vi "3_1_Face_Detection_Inference(CPU,GPU,RT)(Cam).vi"() -> ()   [LabVIEW 2020]
doc: "This example demonstrates the usage of the \"DeepLTK FPGA Addon\" for deploying a Face Detection model on a PXI-FPGA board, utilizing an input image sourced from a camera. \n\nMore Examples: https://github.com/ngenehub/deepltk_fpga_examples"
uses:
  <vilib>/Ngene/Deep Learning Toolkit/Toolkit/NN_Network/Controls/NN_Device.ctl
  <vilib>/vision/driver/IMAQdx.llb/IMAQdx Camera Control Mode.ctl
  <vilib>/Ngene/Deep Learning Toolkit/Toolkit/NN_Network/Controls/NN_Save_Before_Destroy_Options.ctl
  <vilib>/vision/driver/IMAQdx.llb/IMAQdx Buffer Number Mode.ctl
  94985df4-208a-4d6b-b1ec-530e3fcff878.vi
  <vilib>/Ngene/Deep Learning Toolkit/Toolkit/NN_Network/API/NN_Set_Input/3D/NN_Set_Input(3D_SGL_idx).vi
  <vilib>/Ngene/Deep Learning Toolkit/Toolkit/Deep_Learning_Toolkit_by_Ngene.lvlib
  <vilib>/vision/NI_Vision_Development_Module.lvlib
  <vilib>/vision/driver/NI_Vision_Acquisition_Software.lvlib
  <resource>/objmgr/imaqdx.rc
  <vilib>/ptbypt/NI_PtbyPt.lvlib
panel:
  in  "NN_Device":T1
  out "Inference time":dbl=0.10057269999997516 format="%#_4p"
  out "Loop time":dbl=0.10057269999997516 format="%#_4p"
  in  "Camera Resolution":i32(listbox)
  out "Display":T2(plugin-control)
  in  "Confidence_Thresh":sgl=0.19999999
  in  "IOU_Thresh":sgl=0.3
  in  "Camera":refnum<k21>="cam0" caption="IMAQdx Session"
  in  "Weight File Path":path=path "D:/Ngene/GitHub/deepltk_fpga_examples/2_Face_Detection(PXI,sbRIO)/Models/Face_Detection_Original/Face_Detection.bin"
  in  "Configuration File Path":path=path "D:/Ngene/GitHub/deepltk_fpga_examples/2_Face_Detection(PXI,sbRIO)/Models/Face_Detection_Original/Face_Detection.cfg"
  in  "Stop":bool
  # "Overview:  This example demonstrates usage of Deep Learning Toolkit for deploying a Face Detection model, utilizing an input image sourced from a camera.\nThis VI can also be executed on RT targets.\nRequirements: \n•DeepLTK - Deep Learning Toolkit for LabVIEW (https://www.ngene.co/deep-learning-toolkit-for-labview)\n• NI Vision Development Module\n• Web Camera"
  # "Instructions:\nNote: To run the example on an RT target, copy the pretrained model to the RT target.\n1. Provide the \"Network Configuration File Path\" and \"Weight File Path\" locted in \"Models\\Face_Detection_Original\" folder in the project.\n2.\tSelect the camera from \"Camera\" control.\n3.\tUse NN_Device to specify the device (CPU or GPU) for execution. GPU is applicable only for 64-bit LabVIEW.\n4.\tRun the VI. \n5.\t Observe the detections drawn on the \"Display\". The info on the top left of each bounding box represents detected object class and the confidence level.  \n \nMore Examples: https://github.com/ngenehub/deepltk_fpga_examples"
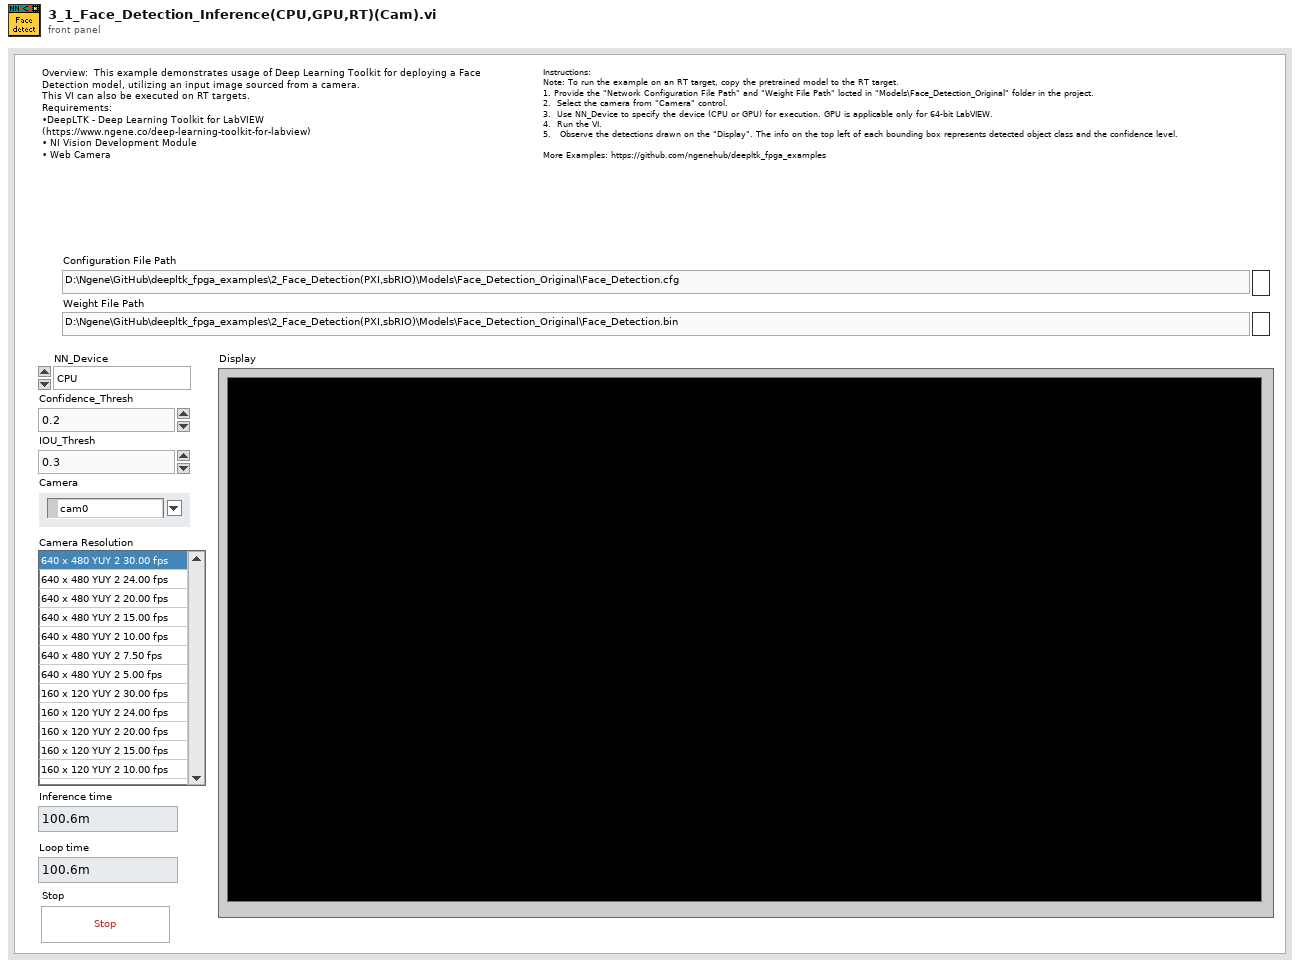
[diagram p1: front panel]
types:
  T1 = typedef "Deep_Learning_Toolkit_by_Ngene.lvlib/NN_Device.ctl" = enum16{"CPU", "GPU"}
  T2 = typedef "IMAQ Image.ctl" = refnum<image>
  T3 = typedef "Deep_Learning_Toolkit_by_Ngene.lvlib/NN_Save_Before_Destroy_Options.ctl" = cluster{"CFG?":bool, "Weights?":bool, "Render?":bool}
  T4 = typedef "NI_Vision_Acquisition_Software.lvlib/IMAQdx Camera Control Mode.ctl" = enum32{"Controller", "Listener"}
  T5 = typedef "Image Type" = u32
  T6 = typedef "IMAQdx.ctl" = refnum<k21>
  T7 = typedef "Deep_Learning_Toolkit_by_Ngene.lvlib/NN_Config_Params.ctl" = cluster{"Name":string, "mBatch":i32, "NN_Train_Params":T8, "LR_Decay_Policy":T11, "Labels":string[], "Loss":T13}
  T8 = typedef "Deep_Learning_Toolkit_by_Ngene.lvlib/NN_Train_Params.ctl" = cluster{"Optimizer":T9, "Beta_1":sgl, "Beta_2":sgl, "Weight Decay(L1)":sgl, "Weight Decay(L2)":sgl, "Data_Sampling":T10}
  T9 = typedef "Deep_Learning_Toolkit_by_Ngene.lvlib/NN_Train_Optimizer.ctl" = enum16{"SGD", "Adam", "Adagrad", "Adadelta", "RMSProp", "Nesterov"}
  T10 = typedef "Deep_Learning_Toolkit_by_Ngene.lvlib/NN_Train_Data_Sampling.ctl" = enum16{"Random", "Sequential"}
  T11 = typedef "Deep_Learning_Toolkit_by_Ngene.lvlib/NN_LR_Policy_Cfg.ctl" = cluster{"Policy_Type":T12, "LR0":dbl, "k":sgl, "WarmUp_Policy":enum16{"Step", "Ramp"}, "WarmUp_Iter":i32, "WarmUp_Ratio":sgl}
  T12 = typedef "Deep_Learning_Toolkit_by_Ngene.lvlib/NN_LR_Policy_Type.ctl" = enum16{"Manual", "Step", "Exp", "1/t"}
  T13 = typedef "Deep_Learning_Toolkit_by_Ngene.lvlib/NN_Loss_Config_Params.ctl" = cluster{"Loss_Type":T14, "Loss_Conf_Params":variant}
  T14 = typedef "Deep_Learning_Toolkit_by_Ngene.lvlib/NN_Loss_Type.ctl" = enum16{"None", "MSE", "CrossEntropy", "YOLO_v2", "YOLO_v4"}
  T15 = typedef "Deep_Learning_Toolkit_by_Ngene.lvlib/NN_Layer_Config_Params.ctl" = cluster{"Layer_Type":T16, "Layer_Conf_Params":variant, "Input Layers":string[]}
  T16 = typedef "Deep_Learning_Toolkit_by_Ngene.lvlib/NN_Layer_Type.ctl" = enum16{"Input1D", "Input3D", "Conv1D", "Conv2D", "Conv2D_Adv", "MaxPool", "AvgPool", "UpSample", "DropOut3D", "ShortCut", "Concat", "SoftMax3D", "FC", "DropOut", "Softmax", "Flatten", "YOLO_v2", "YOLO_v4", "Activation", "BatchNormalization", "Unsupported"}
  T17 = typedef "Deep_Learning_Toolkit_by_Ngene.lvlib/NN.ctl" = cluster{"Name":string, "No of Layers":i32, "mBatch":i32, "Layers":T18[], "Dimty":T19, "Dims_In":T20, "Dims_Out":T20, "Working_Dir":path, "Train?":bool, "Train_Params":T8, "LR_Update_Policy":T11, "Session Data":T21, "Ground_truth":T22, "NNg_hdls":T23, "NN_Device":T1, "GPU Id":i32, "Labels":string[], "Receptive Field":T24[], "Loss_Type":T14, "Loss_Cfg_Prms":variant, "NNG_WS":T25}
  T18 = typedef "Deep_Learning_Toolkit_by_Ngene.lvlib/NN_Layer_ref.ctl" = refnum<data-value>
  T19 = typedef "Deep_Learning_Toolkit_by_Ngene.lvlib/NN_In_Out_Dim-ty.ctl" = enum8{"In1D_Out1D", "In3D_Out1D", "In3D_Out3D", "In3D_OutBBox"}
  T20 = typedef "Deep_Learning_Toolkit_by_Ngene.lvlib/NN_Dims(C,H,W).ctl" = cluster{"C":i32, "H":i32, "W":i32}
  T21 = typedef "Deep_Learning_Toolkit_by_Ngene.lvlib/NN_Train_Session_Data.ctl" = cluster{"Epochs":sgl, "Tot_Iter":i32, "LR":sgl, "LR_iter":i32}
  T22 = typedef "Deep_Learning_Toolkit_by_Ngene.lvlib/NN_Ground_truth.ctl" = cluster{"Y":variant}
  T23 = typedef "Deep_Learning_Toolkit_by_Ngene.lvlib/nng_cuda_handles.ctl" = cluster{"cudnn":u64, "cublas":u64, "stream":u64, "curand":u64}
  T24 = typedef "Deep_Learning_Toolkit_by_Ngene.lvlib/NN_Dims(V,H).ctl" = cluster{"V":i32, "H":i32}
  T25 = typedef "Deep_Learning_Toolkit_by_Ngene.lvlib/NNG_WS.ctl" = cluster{"NNG_WS_Mem":T26, "Max_WS_Size":i64}
  T26 = typedef "Deep_Learning_Toolkit_by_Ngene.lvlib/NNg_WS_Mem_DVR.ctl" = refnum<data-value>
  T27 = typedef "NI_Vision_Acquisition_Software.lvlib/IMAQdx Buffer Number Mode.ctl" = enum32{"Next", "Last", "Buffer Number", "Every", "Last New"}
  T28 = typedef "Deep_Learning_Toolkit_by_Ngene.lvlib/NN_Layer.ctl" = cluster{"Name":string, "Layer_Data":variant, "Layer_Type":T16, "Dims_In":T20, "Layers_In":variant, "Dims_Out":T20, "Layers_Out":variant, "Metrics":T29, "GPU_Data":variant, "mBatch":i32, "NN_Device":T1, "NNg_hdls":T23, "Train?":bool, "Dimty":T30, "RecptField":T31}
  T29 = typedef "Deep_Learning_Toolkit_by_Ngene.lvlib/NN_Layer_Metrics.ctl" = cluster{"Data":dbl, "Params":dbl, "Ops":dbl}
  T30 = typedef "Deep_Learning_Toolkit_by_Ngene.lvlib/NN_Layer_Dimty.ctl" = enum16{"1D", "3D"}
  T31 = typedef "Deep_Learning_Toolkit_by_Ngene.lvlib/NN_Layer_RF_State.ctl" = cluster{"Dims":T24, "J":T24}
  T32 = typedef "Deep_Learning_Toolkit_by_Ngene.lvlib/NN_BBox_Detection.ctl" = cluster{"Class":i32, "Conf Level":sgl, "BBox":T33}
  T33 = typedef "Deep_Learning_Toolkit_by_Ngene.lvlib/NN_BBox.ctl" = cluster{"x":sgl, "y":sgl, "w":sgl, "h":sgl}
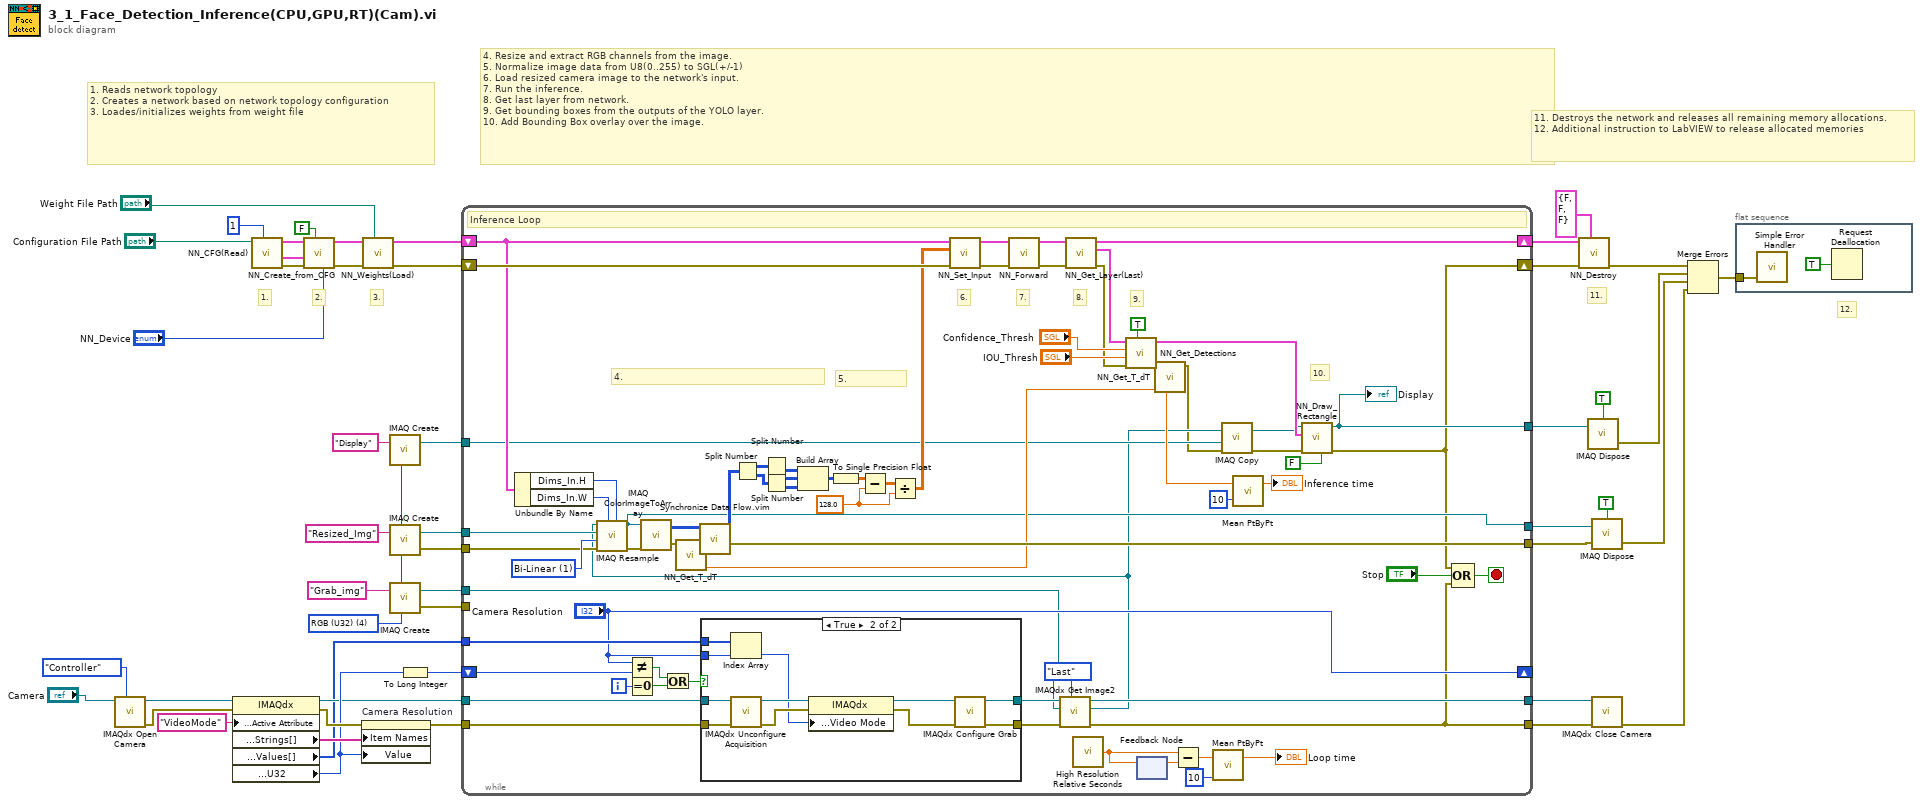
[diagram p0: block diagram]
diagram:
  w2 = T5 4 items=["Grayscale (U8)", "Grayscale (I16)", "Grayscale (SGL)", "Complex (CSG)", "RGB (U32)", "HSL (U32)", "RGB (U64)", "Grayscale (U16)"] ("Image Type")
  # "12."
  # "11.\tDestroys the network and releases all remaining memory allocations.\n12.\tAdditional instruction to LabVIEW to release allocated memories"
  # "11."
  # "4.\tResize and extract RGB channels from the image.\n5.\tNormalize image data from U8(0..255) to SGL(+/-1)\n6.\tLoad resized camera image to the network's input.\n7.\tRun the inference.\n8.\tGet last layer from network.\n9.\tGet bounding boxes from the outputs of the YOLO layer. \n10.\tAdd Bounding Box overlay over the image."
  # "1.\tReads network topology\n2.\tCreates a network based on network topology configuration\n3.\tLoades/initializes weights from weight file"
  # "3."
  # "2."
  # "1."
  n1 = call <vilib>:"IMAQdx Open Camera.vi"("Camera Control Mode"=IMAQdx_Camera_Control_Mode."Controller", "Session In"="Camera") -> ("error out"=w26:errorcluster, "Session Out"=w28:T6)  [unwired: 1 in, 7 out]
  n2 = property class="IMAQdx"(reference=w28, error in=w26, "Camera Attributes:Active Attribute"="VideoMode" ("ActiveAttribute")) -> (reference out=w22:T6, error out=w25:errorcluster, "Camera Attributes:Enum:Strings[]"=w24:string[], "Camera Attributes:Enum:Values[]"=w20:u32[], "Camera Attributes:Value:U32"=w23:u32)
  n3 = call <vilib>:"NN_CFG(Read).vi"("mBatch"=1, "CFG file path"="Configuration File Path") -> ("error out"=w46:errorcluster, "Net_Cfg"=w13:T7, "Layer_Cfg"=w47:T15[])  [unwired: 7 in]
  n4 = call <vilib>:"NN_Create_from_CFG.vi"("NN_Device"="NN_Device", "Train? (false)"=FALSE ("Train?"), "error in (no error)"=w46, "Net_Cfg"=w13, "Layer_Cfg"=w47) -> ("error out"=w45:errorcluster, "NN out"=w44:T17)  [unwired: 5 in]
  n5 = property on="Camera Resolution" class="LstBox (strict)"(error in=w25, "Item Names"=w24, "Value"=w23) -> (error out=w19:errorcluster)  [unwired: 1 in, 1 out]
  n6 = call <vilib>:"NN_Weights(Load).vi"("Weight File Path"="Weight File Path", "error in (no error)"=w45, "NN in"=w44) -> ("error out"=w8:errorcluster, "NN out"=w9:T17)  [unwired: 7 in]
  n7 = call "IMAQ Create"("Image Name"="Display", "Image Type"=w2) -> ("New Image"=w1:T2)  [unwired: 3 in, 1 out]
  n8 = call "IMAQ Create"("Image Name"="Resized_Img", "Image Type"=w2) -> ("New Image"=w34:T2, "error out"=w33:errorcluster)  [unwired: 3 in]
  n9 = call "IMAQ Create"("Image Name"="Grab_img", "Image Type"=w2) -> ("New Image"=w38:T2, "error out"=w41:errorcluster)  [unwired: 3 in]
  n10 = To Long Integer(number=w23) -> (32bit integer=w17:i32)
  n11 = while {
    shift-right: [w87] -> w39
    shift-left: w9 -> [w109]
    shift-right: [w49] -> w40
    shift-left: w8 -> [w114]
    tunnel: [w58] -> w42
    tunnel: w41 -> [_]
    tunnel: w38 -> [w54]
    tunnel: w34 -> [w110]
    tunnel: w33 -> [w100]
    tunnel: [w71] -> w32
    tunnel: [w60] -> w31
    tunnel: w22 -> [w98]
    tunnel: [w97] -> w21
    tunnel: w20 -> [w92]
    tunnel: w19 -> [w91]
    shift-right: ["Camera Resolution"] -> _
    shift-left: w17 -> [w90]
    tunnel: [w82] -> w11
    tunnel: w1 -> [w56]
    i -> [w88]
    stop <- w116 stop-if-true
    w74 = sgl 128.0
    w111 = u32 1 items=["Zero Order", "Bi-Linear", "Quadratic", "Cubic Spline"] ("Interpolation Type")
    # "10."
    # "9."
    # "8."
    # "7."
    # "6."
    # "4."
    # "5."
    # "Inference Loop"
    n12 = Unbundle By Name(w109) -> ("Dims_In.H"=w108:i32, "Dims_In.W"=w107:i32)
    n13 = Not Equal?(x="Camera Resolution", y=w90) -> (x != y?=w95:bool)
    n14 = Equal To 0?(x=w88) -> (x = 0?=w94:bool)
    n15 = Or(x=w95, y=w94) -> (x .or. y?=w96:bool)
    n16 = case shown="True" w96 {
      tunnel: w98 -> [w120 w129]
      tunnel: w91 -> [w119 w128]
      tunnel: [w120 w125] -> w93
      tunnel: [w119 w126] -> w53
      tunnel: w92 -> [_ w131]
      tunnel: "Camera Resolution" -> [_ w130]
      frame False {
      }
      frame True {
        n17 = Index Array(array=w131, index=w130) -> (element=w121:u32)
        n18 = call <vilib>:"IMAQdx Unconfigure Acquisition.vi"("error in"=w128, "Session In"=w129) -> ("error out"=w122:errorcluster, "Session Out"=w127:T6)  [unwired: 8 out]
        n19 = property class="IMAQdx"(reference=w127, error in=w122, "Acquisition Attributes:Video Mode"=w121) -> (reference out=w124:T6, error out=w123:errorcluster)
        n20 = call <vilib>:"IMAQdx Configure Grab.vi"("error in"=w123, "Session In"=w124) -> ("error out"=w126:errorcluster, "Session Out"=w125:T6)  [unwired: 2 in, 6 out]
      }
    }
    n21 = call <vilib>:"IMAQdx Get Image2.vi"("Buffer Number Mode (Next)"=IMAQdx_Buffer_Number_Mode."Last", "error in"=w53, "Image In"=w54, "Session In"=w93) -> ("error out"=w82:errorcluster, "Image Out"=w52:T2, "Session Out"=w97:T6)  [unwired: 4 in, 1 out]
    n22 = call "IMAQ Resample"("X Resolution"=w108, "Y Resolution"=w107, "error in (no error)"=w100, "Interpolation Type"=w111, "Image Dst"=w110, "Image Src"=w52) -> ("error out"=w99:errorcluster, "Image Dst Out"=w60:T2)  [unwired: 4 in]
    n23 = call "IMAQ ColorImageToArray"("Image"=w60, "error in (no error)"=w99) -> ("Image Pixels (U32)"=w73:u32[][], "error out"=w72:errorcluster)  [unwired: 2 in, 1 out]
    n24 = call <vilib>:"NN_Get_T_dT.vi"("error in (no error)"=w72) -> ("T_out"=w66:dbl, "error out"=w70:errorcluster)  [unwired: 6 in, 1 out]
    n25 = call "Synchronize Data Flow.vim"("input 3"=w70, "input 1"=w73) -> ("output 3"=w71:errorcluster, "output 1"=w69:u32[][])  [unwired: 2 in, 2 out]
    n26 = Split Number(x=w69) -> (hi(x)=w102:u16[][], lo(x)=w101:u16[][])
    n27 = Split Number(x=w102) -> (lo(x)=w103:u8[][])  [unwired: 1 out]
    n28 = Split Number(x=w101) -> (hi(x)=w104:u8[][], lo(x)=w105:u8[][])
    n29 = Build Array(w103, w104, w105) -> (w106:u8[][][])
    n30 = To Single Precision Float(number=w106) -> (single precision float=w79:sgl[][][])
    n31 = Subtract(x=w79, y=w74) -> (x-y=w84:sgl[][][])
    n32 = Divide(x=w84, y=w74) -> (x/y=w75:sgl[][][])
    n33 = call-poly <vilib>:"NN_Set_Input.vi"("error in (no error)"=w114, "Data_In(3D_SGL)"=w75, "NN in"=w109) -> ("error out"=w112:errorcluster, "NN out"=w113:T17)  [unwired: 7 in]
    n34 = call <vilib>:"NN_Forward.vi"("error in (no error)"=w112, "NN in"=w113) -> ("error out"=w85:errorcluster, "NN out"=w86:T17)  [unwired: 6 in, 2 out]
    n35 = call <vilib>:"NN_Get_Layer(Last).vi"("error in (no error)"=w85, "NN in"=w86) -> ("error out"=w68:errorcluster, "Last_Layer"=w83:T28, "NN out"=w87:T17)  [unwired: 6 in, 1 out]
    n36 = call <vilib>:"High Resolution Relative Seconds.vi"() -> ("relative seconds"=w117:dbl)
    n37 = call <vilib>:"NN_Get_Detections.vi"("Temporal Averaging (F)"=TRUE ("Enable Averaging"), "error in"=w68, "IOU_Thrsh"="IOU_Thresh", "Confidence_Thrsh"="Confidence_Thresh", "YOLO_Layer"=w83) -> ("error out"=w67:errorcluster, "Detections"=w80:T32[])  [unwired: 5 in]
    n38 = feedback #1() -> (w118:dbl)  [unwired: 1 in]
    n39 = feedback-in #1(w117) -> ()
    n40 = call <vilib>:"NN_Get_T_dT.vi"("T_in"=w66, "error in (no error)"=w67) -> ("error out"=w51:errorcluster, "dT"=w65:dbl)  [unwired: 5 in, 1 out]
    n41 = Subtract(x=w117, y=w118) -> (x-y=w115:dbl)
    n42 = call <vilib>:"Mean PtByPt.vi"("x"=w115, "sample length"=10) -> ("mean"=→"Loop time":dbl)  [unwired: 2 in, 1 out]
    n43 = call "IMAQ Copy"("error in (no error)"=w51, "Image Dst"=w56, "Image Src"=w52) -> ("error out"=w59:errorcluster, "Image Dst Out"=w55:T2)  [unwired: 3 in]
    n44 = call <vilib>:"Mean PtByPt.vi"("x"=w65, "sample length"=10) -> ("mean"=→"Inference time":dbl)  [unwired: 2 in, 1 out]
    n45 = call "NN_Draw_Rectangle.vi"("Clear"=FALSE, "error in (no error)"=w59, "Draw_Boxes"=w80, "Image_in"=w55) -> ("error out"=w49:errorcluster, "Image_out"=w58:T2)  [unwired: 5 in, 1 out]
    "Display" <- w58
    n46 = Compound Arithmetic op=OR(w49, "Stop", w82) -> (w116:bool)
  }
  n47 = call <vilib>:"NN_Destroy.vi"("Save (T, T, T)"=T3 {"CFG?"=FALSE, "Weights?"=FALSE, "Render?"=FALSE} ("Save_Config"), "error in (no error)"=w40, "NN in"=w39) -> ("error out"=w48:errorcluster)  [unwired: 7 in, 1 out]
  n48 = call "IMAQ Dispose"("All Images? (No)"=TRUE, "Image"=w42) -> ("error out"=w36:errorcluster)  [unwired: 4 in]
  n49 = call "IMAQ Dispose"("All Images? (No)"=TRUE, "Image"=w31, "error in (no error)"=w32) -> ("error out"=w16:errorcluster)  [unwired: 3 in]
  n50 = call <vilib>:"IMAQdx Close Camera.vi"("error in"=w11, "Session In"=w21) -> ("error out"=w18:errorcluster)  [unwired: 9 out]
  n51 = Merge Errors(w48, w36, w16, w18) -> (w37:errorcluster)
  n52 = flat-sequence {
    tunnel: w37 -> [w132]
    frame #0 {
      n53 = call <vilib>:"Simple Error Handler.vi"("error in (no error)"=w132) -> ()  [unwired: 4 in, 5 out]
      n54 = Request Deallocation(TRUE ("flag")) -> ()
    }
  }
